vi "PolyHermite.vi"(1 "n":i32) -> (0 "Hn":dbl[](array[numeric]))   [LabVIEW 2017, in "NI_AALPro.lvlib"]
uses:
  <vilib>/Analysis/NI_AALPro.lvlib
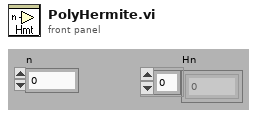
[diagram p1: front panel]
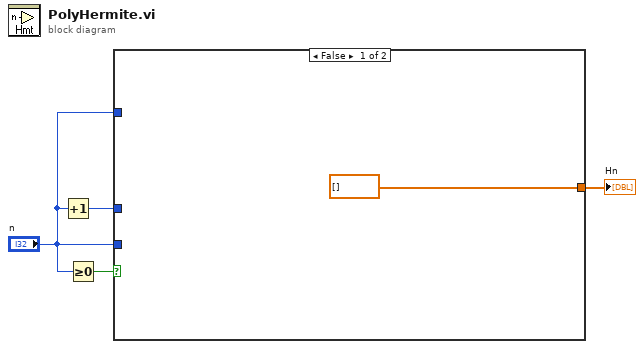
[diagram p0: block diagram]
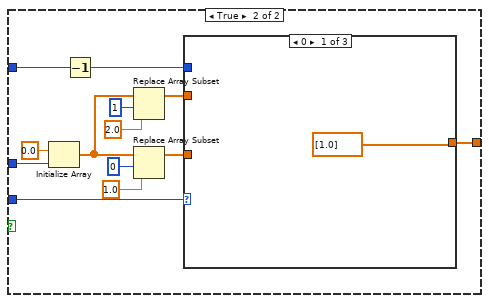
[diagram p2: hidden frame]
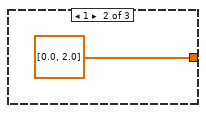
[diagram p3: hidden frame]
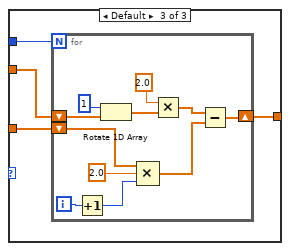
[diagram p4: hidden frame]
diagram:
  n1 = Increment(x="n") -> (x+1=w3:i32)
  n2 = Greater Or Equal To 0?(x="n") -> (x >= 0?=w4:bool)
  n3 = case shown="False" w4 {
    tunnel: "n" -> [_ w18]
    tunnel: w3 -> [_ w9]
    tunnel: "n" -> [_ w7]
    tunnel: [dbl[] [] ("Tn(x)") w8] -> w1
    frame False {
    }
    frame True {
      n4 = Initialize Array(0.0 ("element"), w9) -> (w15:dbl[])
      n5 = Decrement(x=w7) -> (x-1=w6:i32)
      n6 = Replace Array Subset(array=w15, new element=2.0 ("new element/subarray"), index=1) -> (w11:dbl[])
      n7 = Replace Array Subset(array=w15, new element=1.0 ("new element/subarray"), index=0) -> (w10:dbl[])
      n8 = case shown="0" w18 {
        tunnel: w11 -> [_ _ w24]
        tunnel: w10 -> [_ _ w23]
        tunnel: w6 -> [_ _ w22]
        tunnel: [dbl[] [1.0] ("Tn(x)") dbl[] [0.0, 2.0] ("Tn(x)") w21] -> w8
        frame 0 {
        }
        frame 1 {
        }
        frame Default {
          n9 = for {
            N: w22 -> [_]
            shift-right: [w31] -> w21
            shift-left: w24 -> [w35]
            shift-left: w23 -> [w29]
            i -> [w27]
            n10 = Increment(x=w27) -> (x+1=w25:i32)
            n11 = Rotate 1D Array(1:w35, 2:1 ("n")) -> (0:w33:dbl[])
            n12 = Compound Arithmetic op=MULTIPLY(w29, 2.0, w25) -> (w28:dbl[])
            n13 = Multiply(x=2.0, y=w33) -> (x*y=w30:dbl[])
            n14 = Subtract(x=w30, y=w28) -> (x-y=w31:dbl[])
          }
        }
      }
    }
  }
  "Hn" <- w1
